vi "find alias from UID.vi"(10 "UID":string, 11 "instance data":T1[](array[typedef])) -> (3 "Alias":string)   [LabVIEW 2013, in "NISE_CEF_TreeSerializer.lvlib"]
uses:
  NISE_CEF_TreeSerializer.lvlib
  instance data.ctl
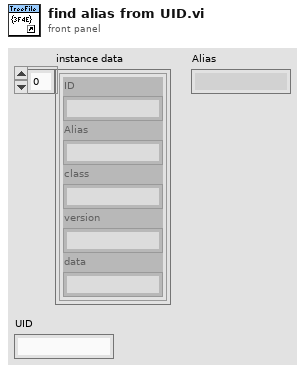
[diagram p1: front panel]
types:
  T1 = typedef "NISE_CEF_TreeSerializer.lvlib/instance data.ctl" = cluster{"ID":string, "Alias":string, "class":string, "version":string, "data":string}
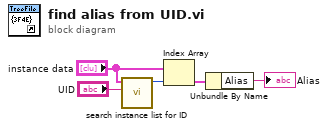
[diagram p0: block diagram]
diagram:
  n1 = call "search instance list for ID.vi"("UID"="UID", "instance data"="instance data") -> ("index"=w3:i32)  [unwired: 9 in]
  n2 = Index Array(array="instance data", index=w3) -> (element=w2:T1)
  n3 = Unbundle By Name(w2) -> ("Alias"=→"Alias":string)
